vi "Destroy Client.vi"(8 "error in (no error)":errorcluster, 11 "gRPC Client in":refnum<class "gRPC Client.lvclass">) -> (0 "error out":errorcluster, 3 "gRPC Client out":refnum<class "gRPC Client.lvclass">)   [LabVIEW 2019, in "gRPC Client (template.proto).lvlib" / "gRPC Client.lvclass"]
uses:
  gRPC Client.lvclass
  gRPC Client.lvclass/gRPC Client.ctl
  Generated_client/Generated_client.lvlib
  <vilib>/gRPC/LabVIEW gRPC Library/Shared/grpcId.ctl
  <vilib>/gRPC/LabVIEW gRPC Library/grpc-lvsupport-release.lvlib
  rsp_Connection Notify.ctl
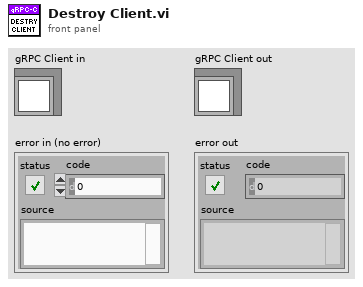
[diagram p1: front panel]
types:
  T1 = typedef "grpc-lvsupport-release.lvlib/grpcId.ctl" = u64
  T2 = typedef "gRPC Client (template.proto).lvlib/gRPC Client.lvclass/rsp_Connection Notify.ctl" = cluster{"gRPC ID":T1, "Connected?":bool}
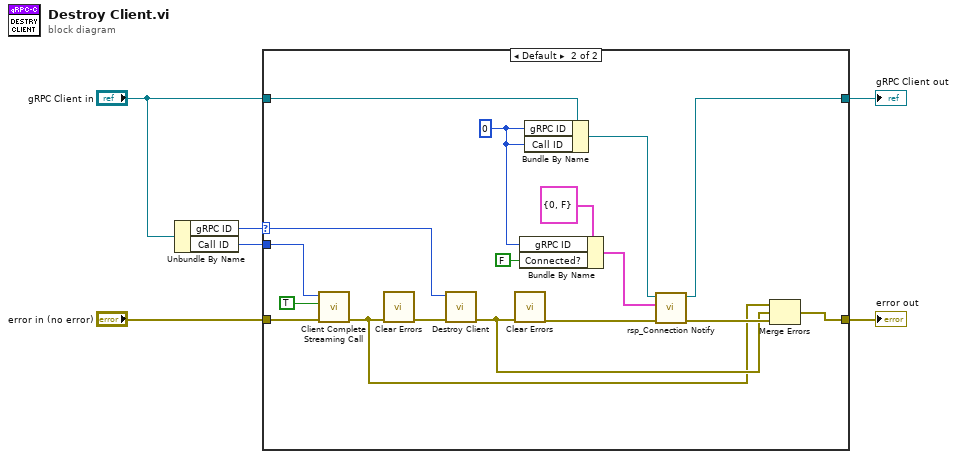
[diagram p0: block diagram]
diagram:
  n1 = Unbundle By Name("gRPC Client in") -> ("gRPC ID"=w5:T1, "Call ID"=w1:T1)
  n2 = case shown="Default" w5 {
    selector: w5 -> [_ w24]
    tunnel: "error in (no error)" -> [w8 w12]
    tunnel: [w8 w14] -> w4
    tunnel: "gRPC Client in" -> [w7 w19]
    tunnel: [w7 w18] -> w2
    tunnel: w1 -> [_ w10]
    frame 0 {
      # "Nothing to do. Connection doesn't exist.\n\nNote: If gRPC ID = 0 (or is invalid) it will cause\nGenerated Client.lvlib : Destroy Client.vi to crash\nand this might crash LabVIEW."
    }
    frame Default {
      w17 = T1 0 ("gRPC ID")
      n3 = call <vilib>:"Client Complete Streaming Call.vi"("error in"=w12, "Cancel All Reads (F)"=TRUE, "Call ID in"=w10) -> ("error out"=w11:errorcluster)  [unwired: 7 in, 1 out]
      n4 = call <vilib>:"Clear Errors.vi"("error in (no error)"=w11) -> ("error out"=w25:errorcluster)  [unwired: 5 in, 1 out]
      n5 = call "Destroy Client.vi"("error in"=w25, "gRPC ID"=w24) -> ("error out"=w13:errorcluster)  [unwired: 9 in]
      n6 = call <vilib>:"Clear Errors.vi"("error in (no error)"=w13) -> ("error out"=w15:errorcluster)  [unwired: 5 in, 1 out]
      n7 = Bundle By Name(cluster=T2 {"gRPC ID"=0, "Connected?"=FALSE} ("Data in"), "gRPC ID"=w17, "Connected?"=FALSE) -> (w21:T2)
      n8 = Bundle By Name(cluster=w19, "gRPC ID"=w17, "Call ID"=w17) -> (w23:refnum<class "gRPC Client.lvclass">)
      n9 = call "rsp_Connection Notify.vi"("error in"=w15, "Data in"=w21, "gRPC Client in"=w23) -> ("error out"=w16:errorcluster, "dup gRPC Client out"=w18:refnum<class "gRPC Client.lvclass">)  [unwired: 7 in]
      n10 = Merge Errors(w11, w13, w16) -> (w14:errorcluster)
    }
  }
  "error out" <- w4
  "gRPC Client out" <- w2
